vi "Default CSV Path.vi"() -> (0 "CSV file path":path)   [LabVIEW 2021, in "Logging.lvlib"]
doc: "Return the default path of the data log file."
uses:
  Logging.lvlib
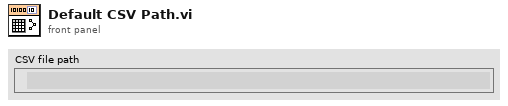
[diagram p1: front panel]
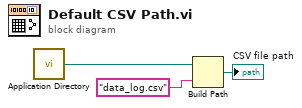
[diagram p0: block diagram]
diagram:
  n1 = call <vilib>:"Application Directory.vi"() -> ("Application Directory"=w1:path)
  n2 = Build Path(base path=w1, name or relative path="data_log.csv") -> (appended path=→"CSV file path":path)
